vi "SRV_Evaluate Sensor Digital_Boolean.vi"(6 "Mask Method (AND)":T1, 9 "Mask":u8 format="%.0b", 11 "Value (U8)":u8 format="%.0b") -> (1 "Result Boolean":bool, 2 "Result":u8 format="%.0b")   [LabVIEW 2009]
uses:
  SRV_Sensor Digital Mask Method.ctl
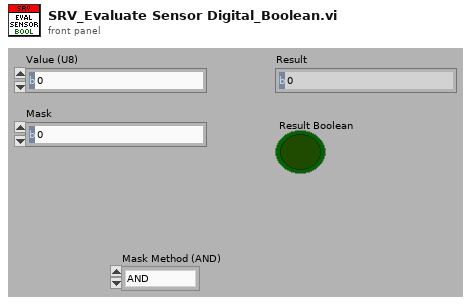
[diagram p1: front panel]
types:
  T1 = typedef "SRV_Sensor Digital Mask Method.ctl" = enum16{"AND", "OR"}
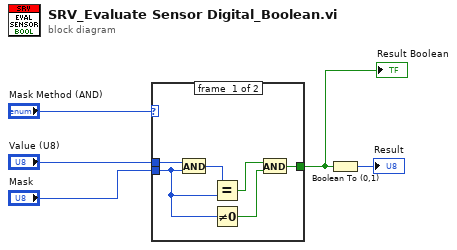
[diagram p0: block diagram]
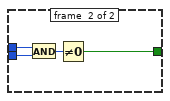
[diagram p2: hidden frame]
diagram:
  n1 = case shown="\"AND\"" "Mask Method (AND)" {
    tunnel: "Value (U8)" -> [w11 w14]
    tunnel: "Mask" -> [w6 w15]
    tunnel: [w8 w12] -> w1
    frame #0 {
      n2 = And(x=w11, y=w6) -> (x .and. y?=w10:u8)
      n3 = Equal?(x=w10, y=w6) -> (x = y?=w9:bool)
      n4 = Not Equal To 0?(x=w6) -> (x != 0?=w7:bool)
      n5 = And(x=w9, y=w7) -> (x .and. y?=w8:bool)
    }
    frame #1 {
      n6 = And(x=w14, y=w15) -> (x .and. y?=w13:u8)
      n7 = Not Equal To 0?(x=w13) -> (x != 0?=w12:bool)
    }
  }
  "Result Boolean" <- w1
  n8 = Boolean To (0,1)(Boolean=w1) -> (0, 1=→"Result":i16)
